vi "z_stack_ OG_waveform.vi"(0 "OG end layer":dbl=10.0, 1 "OG start layer":dbl=8.0, 2 "SPECIFIC scan volt":dbl=5.0, 3 "Steps per volume":dbl=25.0, 4 "OG repitation":dbl=3.0, 6 "Objective线性加速时间":dbl=0.07, 7 "OG Z stack 线性加速 采样信息":cluster{"采样率":dbl, "采样数":dbl}={"采样率"=50000.0, "采样数"=3500.0}, 8 "Objective 刺激steps 时间（s）":dbl=0.033, 9 "OG Z stack 刺激steps 采样信息":cluster{"采样率":dbl, "采样数":dbl}={"采样率"=50000.0, "采样数"=1650.0}, 10 "Objective volet 线性减速 时间（s）":dbl=0.017, 11 "OG Z volet 线性减速 采样信息":cluster{"采样率":dbl, "采样数":dbl}={"采样率"=50000.0, "采样数"=850.0}, 12 "Objective线性减速时间":dbl=0.07, 13 "OG Z stack 线性减速 采样信息":cluster{"采样率":dbl, "采样数":dbl}={"采样率"=50000.0, "采样数"=3500.0}) -> (14 "waveform out":waveform(dbl), 15 "signals 1":waveform(dbl), 16 "signals 2":waveform(dbl), 17 "signals 3":waveform(dbl), 18 "signals 4":waveform(dbl))   [LabVIEW 2018]
uses:
  <vilib>/Waveform/WDTOps.llb/WDT Append Waveforms DBL.vi
  <vilib>/measure/NI_MABase.lvlib
panel:
  out "size(s)":i32
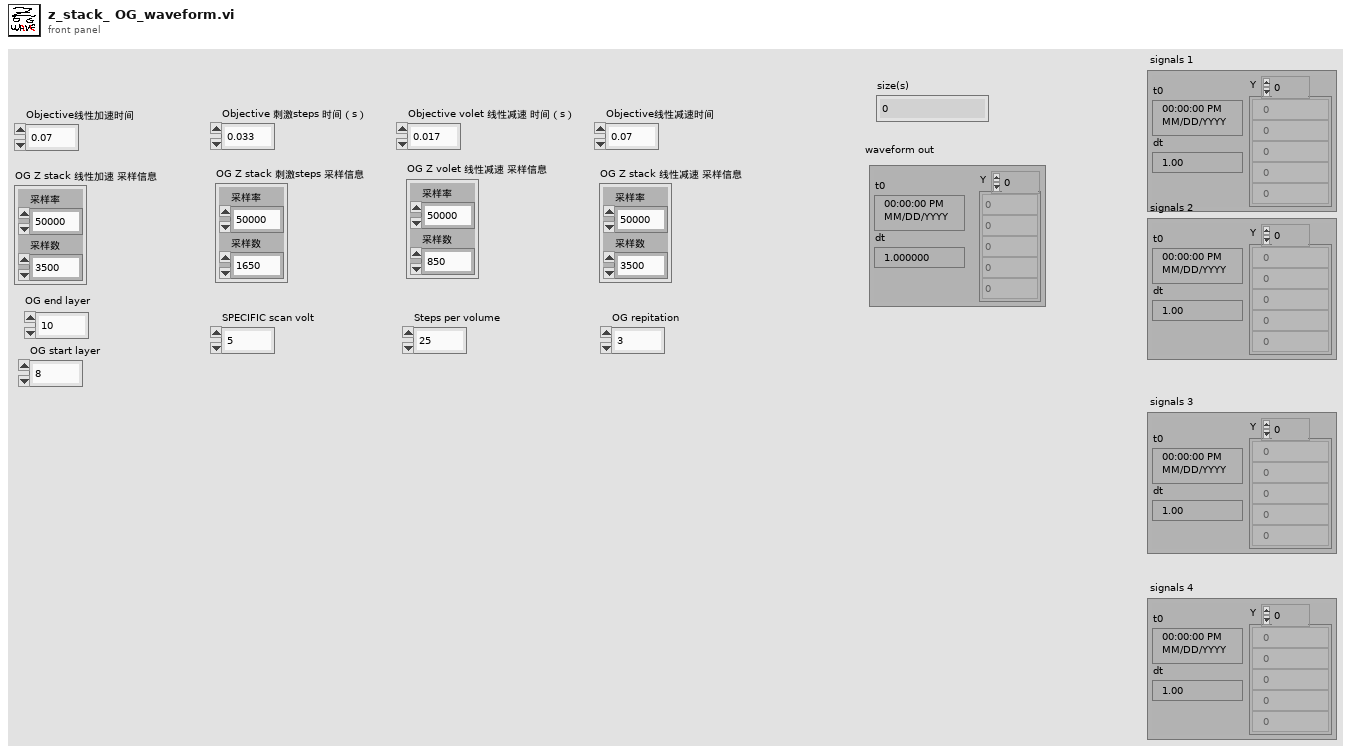
[diagram p1: front panel]
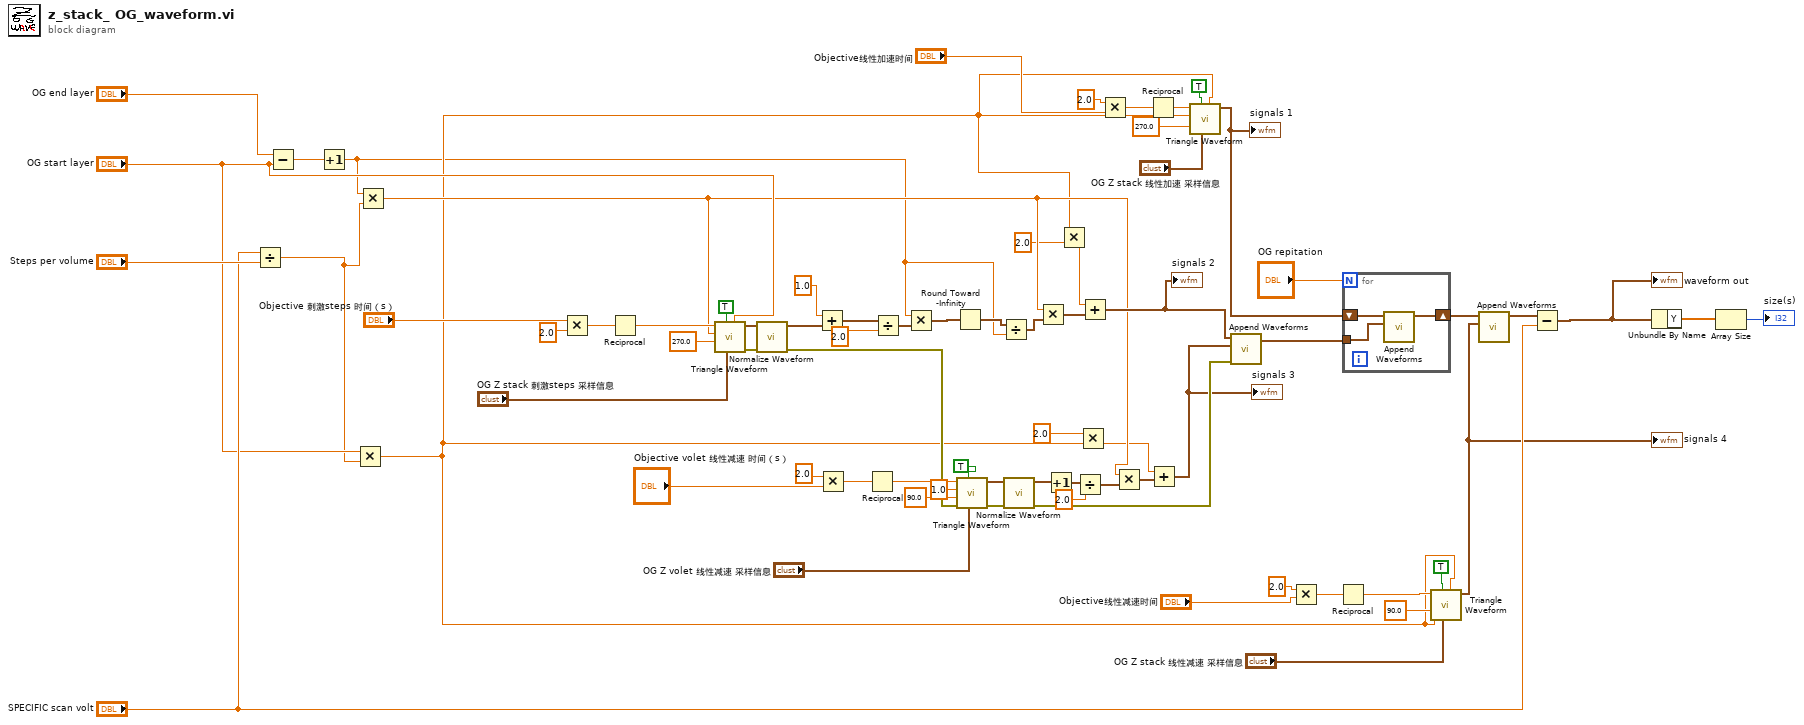
[diagram p0: block diagram]
diagram:
  n1 = Divide(x="SPECIFIC scan volt", y="Steps per volume") -> (x/y=w7:dbl)
  n2 = Subtract(x="OG end layer", y="OG start layer") -> (x-y=w53:dbl)
  n3 = Increment(x=w53) -> (x+1=w5:dbl)
  n4 = Multiply(x="OG start layer", y=w7) -> (x*y=w8:dbl)
  n5 = Multiply(x=w5, y=w7) -> (x*y=w9:dbl)
  n6 = Multiply(x="Objective 刺激steps 时间（s）", y=2.0) -> (x*y=w50:dbl)
  n7 = Reciprocal(x=w50) -> (1/x=w49:dbl)
  n8 = call <vilib>:"Triangle Waveform.vi"("offset"="OG start layer", "sampling info"="OG Z stack 刺激steps 采样信息", "reset signal"=TRUE, "phase"=270.0, "amplitude"=w9, "frequency"=w49) -> ("error out"=w45:errorcluster, "signal out"=w46:waveform(dbl))  [unwired: 4 in]
  n9 = call <vilib>:"Normalize Waveform.vi"("error in (no error)"=w45, "waveform in"=w46) -> ("error out"=w34:errorcluster, "normalized waveform"=w44:waveform(dbl))  [unwired: 6 in, 2 out]
  n10 = Add(x=1.0 ("offset"), y=w44) -> (x+y=w42:waveform(dbl))
  n11 = Multiply(x=2.0 ("y"), y="Objective volet 线性减速 时间（s）") -> (x*y=w37:dbl)
  n12 = Reciprocal(x=w37) -> (1/x=w36:dbl)
  n13 = Divide(x=w42, y=2.0 ("offset")) -> (x/y=w40:waveform(dbl))
  n14 = Multiply(x=w5, y=w40) -> (x*y=w39:waveform(dbl))
  n15 = Round Toward -Infinity(1:w39) -> (0:w6:waveform(dbl))
  n16 = call <vilib>:"Triangle Waveform.vi"("sampling info"="OG Z volet 线性减速 采样信息", "reset signal"=TRUE, "error in (no error)"=w34, "phase"=90.0, "amplitude"=1.0, "frequency"=w36) -> ("error out"=w33:errorcluster, "signal out"=w25:waveform(dbl))  [unwired: 4 in]
  n17 = Divide(x=w6, y=w5) -> (x/y=w10:waveform(dbl))
  n18 = call <vilib>:"Normalize Waveform.vi"("waveform in"=w25) -> ("normalized waveform"=w20:waveform(dbl))  [unwired: 7 in, 3 out]
  n19 = Multiply(x=w9, y=w10) -> (x*y=w17:waveform(dbl))
  n20 = Increment(x=w20) -> (x+1=w22:waveform(dbl))
  n21 = Multiply(x=w8, y=2.0) -> (x*y=w2:dbl)
  n22 = Divide(x=w22, y=2.0) -> (x/y=w23:waveform(dbl))
  n23 = Multiply(x=2.0, y=w8) -> (x*y=w4:dbl)
  n24 = Add(x=w2, y=w17) -> (x+y=w11:waveform(dbl))
  "signals 2" <- w11
  n25 = Multiply(x=2.0 ("y"), y="Objective线性加速时间") -> (x*y=w62:dbl)
  n26 = Multiply(x=w9, y=w23) -> (x*y=w19:waveform(dbl))
  n27 = Reciprocal(x=w62) -> (1/x=w61:dbl)
  n28 = Add(x=w4, y=w19) -> (x+y=w16:waveform(dbl))
  "signals 3" <- w16
  n29 = call <vilib>:"Triangle Waveform.vi"("offset"=w8, "sampling info"="OG Z stack 线性加速 采样信息", "reset signal"=TRUE, "phase"=270.0, "amplitude"=w8, "frequency"=w61) -> ("signal out"=w68:waveform(dbl))  [unwired: 4 in, 1 out]
  "signals 1" <- w68
  n30 = call-poly <vilib>:"Append Waveforms.vi"("error in (no error)"=w33, "waveform B"=w16, "waveform A"=w11) -> ("waveform out"=w65:waveform(dbl))  [unwired: 7 in, 1 out]
  n31 = Multiply(x=2.0 ("y"), y="Objective线性减速时间") -> (x*y=w57:dbl)
  n32 = Reciprocal(x=w57) -> (1/x=w56:dbl)
  n33 = for {
    N: "OG repitation" -> [_]
    shift-right: [w75] -> w64
    shift-left: w68 -> [w74]
    tunnel: w65 -> [w73]
    n34 = call-poly <vilib>:"Append Waveforms.vi"("waveform B"=w73, "waveform A"=w74) -> ("waveform out"=w75:waveform(dbl))  [unwired: 8 in, 1 out]
  }
  n35 = call <vilib>:"Triangle Waveform.vi"("offset"=w8, "sampling info"="OG Z stack 线性减速 采样信息", "reset signal"=TRUE, "phase"=90.0, "amplitude"=w8, "frequency"=w56) -> ("signal out"=w15:waveform(dbl))  [unwired: 4 in, 1 out]
  "signals 4" <- w15
  n36 = call-poly <vilib>:"Append Waveforms.vi"("waveform B"=w15, "waveform A"=w64) -> ("waveform out"=w28:waveform(dbl))  [unwired: 8 in, 1 out]
  n37 = Subtract(x=w28, y="SPECIFIC scan volt") -> (x-y=w12:waveform(dbl))
  "waveform out" <- w12
  n38 = Unbundle By Name(w12) -> ("Y"=w14:dbl[])
  n39 = Array Size(array=w14) -> (size(s)=→"size(s)":i32)
